vi "XML Read ID and Result.vi"(10 "Result Contents":string[](array[string]), 11 "Result Tags":string[](array[string])) -> (2 "Name.Sub":string[](array[string]), 3 "Result ID":i32[](array[numeric]))   [LabVIEW 2011, in "Design Server.lvlib"]
uses:
  Design Server.lvlib
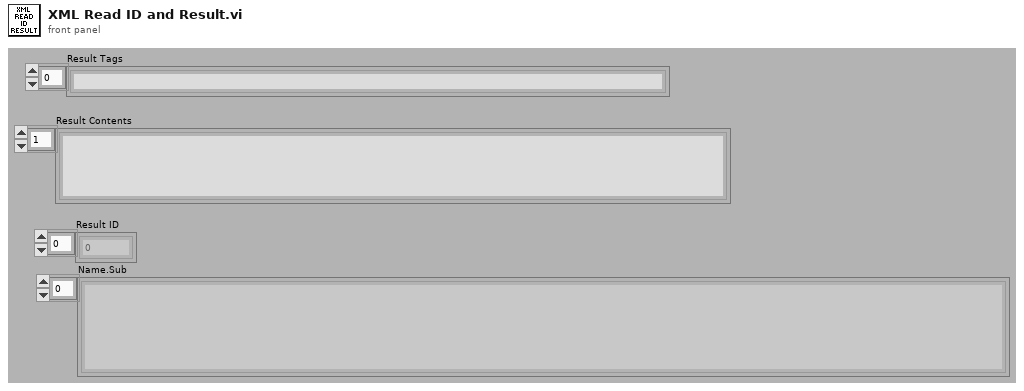
[diagram p1: front panel]
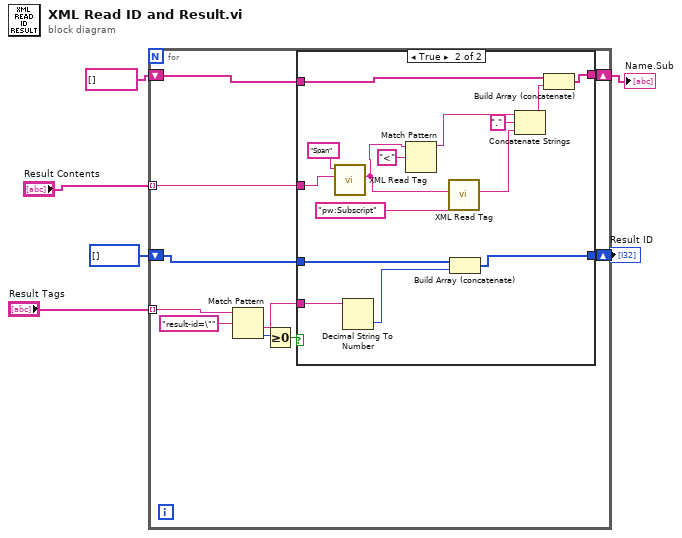
[diagram p0: block diagram]
diagram:
  n1 = for {
    tunnel: "Result Tags" -> [w16] mode=indexing
    shift-right: [w10] -> w5
    shift-left: i32[] [] -> [w11]
    tunnel: "Result Contents" -> [w9] mode=indexing
    shift-right: [w7] -> w1
    shift-left: string[] [] -> [w8]
    n2 = Match Pattern(string=w16, regular expression="result-id=\"") -> (after substring=w12:string, offset past match=w14:i32)  [unwired: 1 in, 2 out]
    n3 = Greater Or Equal To 0?(x=w14) -> (x >= 0?=w13:bool)
    n4 = case shown="True" w13 {
      tunnel: w12 -> [_ w33]
      tunnel: w11 -> [w18 w31]
      tunnel: [w18 w30] -> w10
      tunnel: w9 -> [_ w29]
      tunnel: w8 -> [w17 w27]
      tunnel: [w17 w26] -> w7
      frame False {
      }
      frame True {
        n5 = call "XML Read Tag.vi"("XML"=w29, "XML Tag"="Span") -> ("content"=w19:string)  [unwired: 7 in, 2 out]
        n6 = Decimal String To Number(string=w33) -> (number=w32:i32)  [unwired: 2 in, 1 out]
        n7 = Match Pattern(string=w19, regular expression="<") -> (before substring=w23:string)  [unwired: 1 in, 3 out]
        n8 = call "XML Read Tag.vi"("XML"=w19, "XML Tag"="pw:Subscript") -> ("content"=w21:string)  [unwired: 7 in, 2 out]
        n9 = Build Array (concatenate)(w31, w32) -> (w30:i32[])
        n10 = Concatenate Strings(w23, "." ("string"), w21) -> (w24:string)
        n11 = Build Array (concatenate)(w27, w24) -> (w26:string[])
      }
    }
  }
  "Result ID" <- w5
  "Name.Sub" <- w1
